vi "Mean(DBL).vi"(7 "enable":bool=TRUE, 8 "error in":errorcluster, 9 "reset":bool, 11 "input":dbl) -> (0 "error out":errorcluster, 3 "mean":dbl)   [LabVIEW 2012]
panel:
  out "length":i32
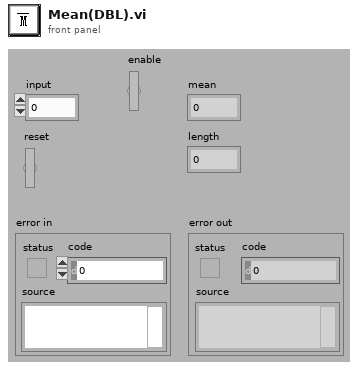
[diagram p1: front panel]
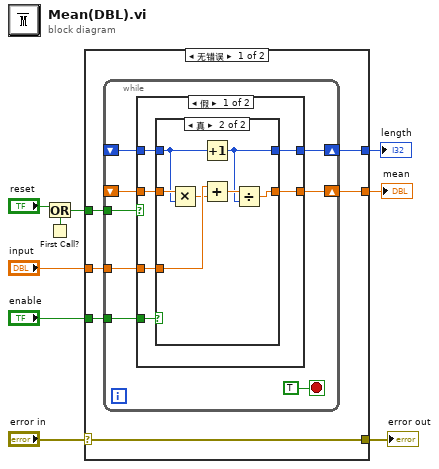
[diagram p0: block diagram]
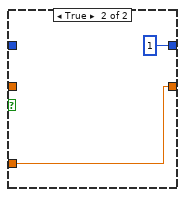
[diagram p3: hidden frame]
diagram:
  n1 = First Call?() -> (First Call?: T/F=w7:bool)
  n2 = Or(x="reset", y=w7) -> (x .or. y?=w5:bool)
  n3 = case shown="无错误" "error in" {
    selector: "error in" -> [w15 w41]
    tunnel: [w15 w41] -> w9
    tunnel: w5 -> [w14 _]
    tunnel: "enable" -> [w13 _]
    tunnel: "input" -> [w12 _]
    tunnel: [w11 _] -> w2
    tunnel: [w10 _] -> w1
    frame No Error {
      n4 = while {
        shift-right: [w21] -> w11
        shift-left: _ -> [w22]
        shift-right: [w20] -> w10
        shift-left: _ -> [w19]
        tunnel: w14 -> [w18]
        tunnel: w13 -> [w17]
        tunnel: w12 -> [w16]
        stop <- TRUE stop-if-true
        n5 = case shown="假" w18 {
          tunnel: [w26 w40] -> w21
          tunnel: w17 -> [w29 _]
          tunnel: w16 -> [w28 w40]
          tunnel: w22 -> [w27 _]
          tunnel: [w24 1] -> w20
          tunnel: w19 -> [w25 _]
          frame False {
            n6 = case shown="真" w29 {
              tunnel: w28 -> [_ w36]
              tunnel: w27 -> [w31 w38]
              tunnel: [w31 w34] -> w26
              tunnel: w25 -> [w30 w37]
              tunnel: [w30 w32] -> w24
              frame False {
              }
              frame True {
                n7 = Multiply(x=w38, y=w37) -> (x*y=w35:dbl)
                n8 = Increment(x=w37) -> (x+1=w32:i32)
                n9 = Add(x=w36, y=w35) -> (x+y=w33:dbl)
                n10 = Divide(x=w33, y=w32) -> (x/y=w34:dbl)
              }
            }
          }
          frame True {
          }
        }
      }
    }
    frame Error {
    }
  }
  "error out" <- w9
  "mean" <- w2
  "length" <- w1
